vi "VisionNetwork.vi"   [LabVIEW 2020]
uses:
  <vilib>/Rock Robotics/Network Tables/NT Read Number.vi
  VisionGlobals.vi
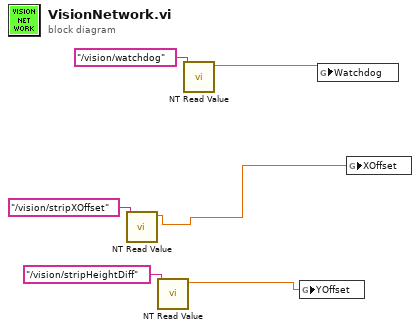
[diagram p0: block diagram]
diagram:
  n1 = call-poly <vilib>:"NT Read Value.vi"("Name"="/vision/stripXOffset") -> ("Numeric"=w3:dbl)  [unwired: 9 in, 1 out]
  n2 = call-poly <vilib>:"NT Read Value.vi"("Name"="/vision/stripHeightDiff") -> ("Numeric"=w4:dbl)  [unwired: 9 in, 1 out]
  n3 = call-poly <vilib>:"NT Read Value.vi"("Name"="/vision/watchdog") -> ("Numeric"=w1:dbl)  [unwired: 9 in, 1 out]
  n4 = global write "VisionGlobals.vi" "YOffset"(w4) -> ()
  n5 = global write "VisionGlobals.vi" "Watchdog"(w1) -> ()
  n6 = global write "VisionGlobals.vi" "XOffset"(w3) -> ()
